vi "Calculate Galvo Control Voltage to Image Size and Max FOV.vi"(8 "Error In":errorcluster, 11 "System Parameters [In]":T1={"Optical Parameters"={"Obj. Focal Length [mm]"=0.0, "Scan Lens EFL[mm]"=0.0, "Tube Lens EFL[mm]"=0.0, "Galvo V Range (+/-)"=0.0, "Galvo Max Half Angle [Deg]"=0.0, "Max Galvo Range[%]"=0.0}, "Vibratome"={"Z Bottom [mm]"=0.0, "Pre Cut Dwell [s]"=0.0, "Blade Frequency [RPM]"=0, "Slice Speed [mm/s]"=0.0, "Post Cut Dwell [s]"=0.0, "Ramp Time [s]"=0.0, "Start X [mm]"=0.0, "Start Y [mm]"=0.0, "Slice Length [mm]"=0.0, "Slice Axis"=enum."Y Axis", "Controller VISA Ref"="COM4", "Blade Frequency [Hz]"=0, "Analog Out Channel"="GalvoCtrl/ao0,GalvoCtrl/ao1", "Pixel Clock Source"="/GalvoCtrl/PFI0"}, "Table Stages"={"X Stage"={"Position"=0.0, "Is.Enabled?"=FALSE, "Is.Connected?"=FALSE, "Device SN"="45876539", "AccelerationMaximum"=0.0, "VelocityMaximum"=0.0, "Acceleration"=0.0, "Velocity"=0.0, "waitTimeout (ms)"=0, "Model"=enum."None", "Is.Homed?"=FALSE, "MOVE"=FALSE}, "Y Stage"={"Position"=0.0, "Is.Enabled?"=FALSE, "Is.Connected?"=FALSE, "Device SN"="45876539", "AccelerationMaximum"=0.0, "VelocityMaximum"=0.0, "Acceleration"=0.0, "Velocity"=0.0, "waitTimeout (ms)"=0, "Model"=enum."None", "Is.Homed?"=FALSE, "MOVE"=FALSE}, "Z Stage"={"Position"=0.0, "Is.Enabled?"=FALSE, "Is.Connected?"=FALSE, "Device SN"="45876539", "AccelerationMaximum"=0.0, "VelocityMaximum"=0.0, "Acceleration"=0.0, "Velocity"=0.0, "waitTimeout (ms)"=0, "Model"=enum."None", "Is.Homed?"=FALSE, "MOVE"=FALSE}}, "Imaging Parameter"={"Raster Scan Direction"=enum."Uni Directional", "Pixel Dwell Time [Clock Cycles]"=0, "Flyback Time [Clock Cycles]"=0, "XY Center [um]"={"X"=1.0, "Y"=1.0}, "Pixel Step Size [um] X"=1.0, "XY Image Size"=enum."256 x 256", "Custom"=FALSE, "Custom Size"={"X"=1, "Y"=1}, "Line Averages"=1, "Pixel Step Size [um] Y"=0.0}, "Galvo HW Parameters"={"Analog Out Channel"="GalvoCtrl/ao0,GalvoCtrl/ao1", "Min Voltage"=-10.0, "Max Voltage"=10.0, "Pixel Clock Source"="/GalvoCtrl/PFI0", "Sample Rate"=1000.0, "Line Clock Out Ch"="GalvoCtrl/port0/line0", "2P ready check"="GalvoCtrl/port0/line0"}, "Alazar parameters"={"Trigger Settings"={"General Trigger Settings"={"Trigger Operation"=0, "Coupling ID"=2, "Range ID"=2, "Delay"=0, "Timeout Ticks"=0, "Mode"=1, "Parameter"=1}, "Trigger Engine 1"={"Trigger Engine"=0, "Source"=2, "Slope"=1, "Level"=140}, "Trigger Engine 2"={"Trigger Engine"=1000, "Source"=4294967295, "Slope"=1, "Level"=2048}}, "Device ID"={"System ID"=1, "Board ID"=1}, "Ch A Input Control"={"Channel"=1, "Coupling"=2, "Range"=10, "Impedance"=2}, "Ch B Input Control"={"Channel"=2, "Coupling"=2, "Range"=10, "Impedance"=2}, "Acq Settings"={"Record Length"=1440, "Offset"=0, "Records Per Buffer"=2048, "Records Count (Records/Acq)"=2147483647, "Window Type"=1, "Footer"=0, "Samples per record"=2048, "Output Format"=257}, "Capture Clock"={"Sample Rate"=100, "Decimation"=0, "Source"=2, "Edge"=0}}, "Mosaic Paramter"={"X Axis"={"Start [mm]"=0.0, "Steps [pts]"=0.0, "End [mm]"=0.0}, "Y Axis"={"Start [mm]"=0.0, "Steps [pts]"=0.0, "End [mm]"=0.0}, "Scan Pattern"=enum."Uni-directional", "Overlap Options"={"Overlap Type"=enum."No Overlap", "Percent Overlap"=0, "Justify"=enum."Start"}}, "Manual Controls"={"Z0"=10.0, "First image height"=0.0, "Data Path"=path "", "Save parameters"={"start pixel"=45, "#pixels to save"=100}, "Center Galvos"=FALSE, "Acquisition mode"=enum."Alazar FFT", "PSOCT Channel"=1, "Save"=FALSE, "AIP rotation angle"=0.0, "ret ds"=FALSE, "Pause?"=FALSE, "Outgoing Mail Server (SMTP)"="smtp.gmail.com", "Email"="", "Password"="", "Carrier 1"=enum."Sprint", "phone number 1"="", "Subject"="", "Message"="", "blocker position"=enum."every two slices", "Carrier 2"=enum."Sprint", "phone number 2"="", "tissue boundary"=FALSE, "Threshold"=0.0}, "Vibratome Axis"={"Start [mm](first cut height)"=45.85, "slice thickness[um]"=2.1, "#slice"=111, "image thickness(um)"=0.0, "#images"=0, "30um?"=FALSE}} {"Manual Controls"."PSOCT Channel" items=["A"=1, "B"=2, "A + B"=3, "C"=4, "A + C"=5, "A + B"=6, "D"=8, "A + D"=9, "B + D"=10, "C + D"=12, "A + B + C + D"=15]; "Alazar parameters"."Capture Clock"."Edge" items=["Rising", "Falling"]; "Alazar parameters"."Capture Clock"."Source" items=["Internal"=1, "Fast External"=2, "Medium External"=3, "Slow External"=4, "External AC"=5, "External DC"=6, "External 10MHz"=7]; "Alazar parameters"."Acq Settings"."Output Format" items=["Float Log"=11, "Float Amp"=10, "U16_LOG"=1, "U16_AMP2"=257, "Real"=3, "Imag"=4]; "Alazar parameters"."Acq Settings"."Footer" items=["FOOTER_NONE", "FOOTER_NPT"]; "Alazar parameters"."Acq Settings"."Window Type" items=["DSP_WINDOW_NONE", "DSP_WINDOW_HANNING", "DSP_WINDOW_HAMMING", "DSP_WINDOW_BLACKMAN", "DSP_WINDOW_BLACKMAN_HARRIS", "DSP_WINDOW_BARTLETT"]; "Alazar parameters"."Ch B Input Control"."Channel" items=["A"=1, "B"=2, "C"=4, "D"=8]; "Alazar parameters"."Ch B Input Control"."Coupling" items=["AC"=1, "DC"=2]; "Alazar parameters"."Ch B Input Control"."Range" items=["20 mV"=1, "40 mV"=2, "50 mV"=3, "80 mV"=4, "100 mV"=5, "200 mV"=6, "400 mV"=7, "500 mV"=8, "800 mV"=9, "1 V"=10, "1.25 V"=33, "2 V"=11, "4 V"=12, "5 V"=13, "8 V"=14, "10 V"=15, "20 V"=16]; "Alazar parameters"."Ch B Input Control"."Impedance" items=["1 MOhm"=1, "50 Ohm"=2, ""=0]; "Alazar parameters"."Ch A Input Control"."Channel" items=["A"=1, "B"=2, "C"=4, "D"=8]; "Alazar parameters"."Ch A Input Control"."Coupling" items=["AC"=1, "DC"=2]; "Alazar parameters"."Ch A Input Control"."Range" items=["20 mV"=1, "40 mV"=2, "50 mV"=3, "80 mV"=4, "100 mV"=5, "200 mV"=6, "400 mV"=7, "500 mV"=8, "800 mV"=9, "1 V"=10, "1.25 V"=33, "2 V"=11, "4 V"=12, "5 V"=13, "8 V"=14, "10 V"=15, "20 V"=16]; "Alazar parameters"."Ch A Input Control"."Impedance" items=["1 MOhm"=1, "50 Ohm"=2, ""=0]; "Alazar parameters"."Trigger Settings"."General Trigger Settings"."Trigger Operation" items=["J", "K", "J OR K", "J AND K", "J XOR K", "J AND NOT K", "NOT J AND K"]; "Alazar parameters"."Trigger Settings"."General Trigger Settings"."Coupling ID" items=["AC"=1, "DC"=2]; "Alazar parameters"."Trigger Settings"."General Trigger Settings"."Range ID" items=["5 V", "1 V", "TTL"]; "Alazar parameters"."Trigger Settings"."Trigger Engine 1"."Trigger Engine" items=["J", "K"]; "Alazar parameters"."Trigger Settings"."Trigger Engine 1"."Source" items=["A", "B", "External", "Disable", "C", "D"]; "Alazar parameters"."Trigger Settings"."Trigger Engine 1"."Slope" items=["Positive"=1, "Negative"=2]; "Alazar parameters"."Trigger Settings"."Trigger Engine 2"."Trigger Engine" items=["J", "K"]; "Alazar parameters"."Trigger Settings"."Trigger Engine 2"."Source" items=["A", "B", "External", "Disable", "C", "D"]; "Alazar parameters"."Trigger Settings"."Trigger Engine 2"."Slope" items=["Positive"=1, "Negative"=2]; "Imaging Parameter"."Pixel Step Size [um] Y" min=0.0 max=10.0 step=0.01; "Imaging Parameter"."Line Averages" min=1 max=30 step=1; "Imaging Parameter"."Flyback Time [Clock Cycles]" max=10 step=1; "Imaging Parameter"."Pixel Step Size [um] X" min=0.0 max=10.0 step=0.01; "Imaging Parameter"."Custom Size"."Y" min=1 max=30 step=1; "Imaging Parameter"."Custom Size"."X" min=1 max=30 step=1; "Imaging Parameter"."XY Center [um]"."Y" min=1.0 max=30.0 step=1.0; "Imaging Parameter"."XY Center [um]"."X" min=1.0 max=30.0 step=1.0; "Imaging Parameter"."Pixel Dwell Time [Clock Cycles]" max=10 step=1}) -> (0 "Error Out":errorcluster, 1 "Max Half FOV (um)":dbl, 2 "Galvo [um/V]":dbl, 3 "System Parameters [Out]":T1={"Optical Parameters"={"Obj. Focal Length [mm]"=0.0, "Scan Lens EFL[mm]"=0.0, "Tube Lens EFL[mm]"=0.0, "Galvo V Range (+/-)"=0.0, "Galvo Max Half Angle [Deg]"=0.0, "Max Galvo Range[%]"=0.0}, "Vibratome"={"Z Bottom [mm]"=0.0, "Pre Cut Dwell [s]"=0.0, "Blade Frequency [RPM]"=0, "Slice Speed [mm/s]"=0.0, "Post Cut Dwell [s]"=0.0, "Ramp Time [s]"=0.0, "Start X [mm]"=0.0, "Start Y [mm]"=0.0, "Slice Length [mm]"=0.0, "Slice Axis"=enum."Y Axis", "Controller VISA Ref"="COM4", "Blade Frequency [Hz]"=0, "Analog Out Channel"="GalvoCtrl/ao0,GalvoCtrl/ao1", "Pixel Clock Source"="/GalvoCtrl/PFI0"}, "Table Stages"={"X Stage"={"Position"=0.0, "Is.Enabled?"=FALSE, "Is.Connected?"=FALSE, "Device SN"="45876539", "AccelerationMaximum"=0.0, "VelocityMaximum"=0.0, "Acceleration"=0.0, "Velocity"=0.0, "waitTimeout (ms)"=0, "Model"=enum."None", "Is.Homed?"=FALSE, "MOVE"=FALSE}, "Y Stage"={"Position"=0.0, "Is.Enabled?"=FALSE, "Is.Connected?"=FALSE, "Device SN"="45876539", "AccelerationMaximum"=0.0, "VelocityMaximum"=0.0, "Acceleration"=0.0, "Velocity"=0.0, "waitTimeout (ms)"=0, "Model"=enum."None", "Is.Homed?"=FALSE, "MOVE"=FALSE}, "Z Stage"={"Position"=0.0, "Is.Enabled?"=FALSE, "Is.Connected?"=FALSE, "Device SN"="45876539", "AccelerationMaximum"=0.0, "VelocityMaximum"=0.0, "Acceleration"=0.0, "Velocity"=0.0, "waitTimeout (ms)"=0, "Model"=enum."None", "Is.Homed?"=FALSE, "MOVE"=FALSE}}, "Imaging Parameter"={"Raster Scan Direction"=enum."Uni Directional", "Pixel Dwell Time [Clock Cycles]"=0, "Flyback Time [Clock Cycles]"=0, "XY Center [um]"={"X"=1.0, "Y"=1.0}, "Pixel Step Size [um] X"=1.0, "XY Image Size"=enum."256 x 256", "Custom"=FALSE, "Custom Size"={"X"=1, "Y"=1}, "Line Averages"=1, "Pixel Step Size [um] Y"=0.0}, "Galvo HW Parameters"={"Analog Out Channel"="GalvoCtrl/ao0,GalvoCtrl/ao1", "Min Voltage"=-10.0, "Max Voltage"=10.0, "Pixel Clock Source"="/GalvoCtrl/PFI0", "Sample Rate"=1000.0, "Line Clock Out Ch"="GalvoCtrl/port0/line0", "2P ready check"="GalvoCtrl/port0/line0"}, "Alazar parameters"={"Trigger Settings"={"General Trigger Settings"={"Trigger Operation"=0, "Coupling ID"=2, "Range ID"=2, "Delay"=0, "Timeout Ticks"=0, "Mode"=1, "Parameter"=1}, "Trigger Engine 1"={"Trigger Engine"=0, "Source"=2, "Slope"=1, "Level"=140}, "Trigger Engine 2"={"Trigger Engine"=1000, "Source"=4294967295, "Slope"=1, "Level"=2048}}, "Device ID"={"System ID"=1, "Board ID"=1}, "Ch A Input Control"={"Channel"=1, "Coupling"=2, "Range"=10, "Impedance"=2}, "Ch B Input Control"={"Channel"=2, "Coupling"=2, "Range"=10, "Impedance"=2}, "Acq Settings"={"Record Length"=1440, "Offset"=0, "Records Per Buffer"=2048, "Records Count (Records/Acq)"=2147483647, "Window Type"=1, "Footer"=0, "Samples per record"=2048, "Output Format"=257}, "Capture Clock"={"Sample Rate"=100, "Decimation"=0, "Source"=2, "Edge"=0}}, "Mosaic Paramter"={"X Axis"={"Start [mm]"=0.0, "Steps [pts]"=0.0, "End [mm]"=0.0}, "Y Axis"={"Start [mm]"=0.0, "Steps [pts]"=0.0, "End [mm]"=0.0}, "Scan Pattern"=enum."Uni-directional", "Overlap Options"={"Overlap Type"=enum."No Overlap", "Percent Overlap"=0, "Justify"=enum."Start"}}, "Manual Controls"={"Z0"=10.0, "First image height"=0.0, "Data Path"=path "", "Save parameters"={"start pixel"=45, "#pixels to save"=100}, "Center Galvos"=FALSE, "Acquisition mode"=enum."Alazar FFT", "PSOCT Channel"=1, "Save"=FALSE, "AIP rotation angle"=0.0, "ret ds"=FALSE, "Pause?"=FALSE, "Outgoing Mail Server (SMTP)"="smtp.gmail.com", "Email"="", "Password"="", "Carrier 1"=enum."Sprint", "phone number 1"="", "Subject"="", "Message"="", "blocker position"=enum."every two slices", "Carrier 2"=enum."Sprint", "phone number 2"="", "tissue boundary"=FALSE, "Threshold"=0.0}, "Vibratome Axis"={"Start [mm](first cut height)"=45.85, "slice thickness[um]"=2.1, "#slice"=111, "image thickness(um)"=0.0, "#images"=0, "30um?"=FALSE}} {"Manual Controls"."PSOCT Channel" items=["A"=1, "B"=2, "A + B"=3, "C"=4, "A + C"=5, "A + B"=6, "D"=8, "A + D"=9, "B + D"=10, "C + D"=12, "A + B + C + D"=15]; "Alazar parameters"."Capture Clock"."Edge" items=["Rising", "Falling"]; "Alazar parameters"."Capture Clock"."Source" items=["Internal"=1, "Fast External"=2, "Medium External"=3, "Slow External"=4, "External AC"=5, "External DC"=6, "External 10MHz"=7]; "Alazar parameters"."Acq Settings"."Output Format" items=["Float Log"=11, "Float Amp"=10, "U16_LOG"=1, "U16_AMP2"=257, "Real"=3, "Imag"=4]; "Alazar parameters"."Acq Settings"."Footer" items=["FOOTER_NONE", "FOOTER_NPT"]; "Alazar parameters"."Acq Settings"."Window Type" items=["DSP_WINDOW_NONE", "DSP_WINDOW_HANNING", "DSP_WINDOW_HAMMING", "DSP_WINDOW_BLACKMAN", "DSP_WINDOW_BLACKMAN_HARRIS", "DSP_WINDOW_BARTLETT"]; "Alazar parameters"."Ch B Input Control"."Channel" items=["A"=1, "B"=2, "C"=4, "D"=8]; "Alazar parameters"."Ch B Input Control"."Coupling" items=["AC"=1, "DC"=2]; "Alazar parameters"."Ch B Input Control"."Range" items=["20 mV"=1, "40 mV"=2, "50 mV"=3, "80 mV"=4, "100 mV"=5, "200 mV"=6, "400 mV"=7, "500 mV"=8, "800 mV"=9, "1 V"=10, "1.25 V"=33, "2 V"=11, "4 V"=12, "5 V"=13, "8 V"=14, "10 V"=15, "20 V"=16]; "Alazar parameters"."Ch B Input Control"."Impedance" items=["1 MOhm"=1, "50 Ohm"=2, ""=0]; "Alazar parameters"."Ch A Input Control"."Channel" items=["A"=1, "B"=2, "C"=4, "D"=8]; "Alazar parameters"."Ch A Input Control"."Coupling" items=["AC"=1, "DC"=2]; "Alazar parameters"."Ch A Input Control"."Range" items=["20 mV"=1, "40 mV"=2, "50 mV"=3, "80 mV"=4, "100 mV"=5, "200 mV"=6, "400 mV"=7, "500 mV"=8, "800 mV"=9, "1 V"=10, "1.25 V"=33, "2 V"=11, "4 V"=12, "5 V"=13, "8 V"=14, "10 V"=15, "20 V"=16]; "Alazar parameters"."Ch A Input Control"."Impedance" items=["1 MOhm"=1, "50 Ohm"=2, ""=0]; "Alazar parameters"."Trigger Settings"."General Trigger Settings"."Trigger Operation" items=["J", "K", "J OR K", "J AND K", "J XOR K", "J AND NOT K", "NOT J AND K"]; "Alazar parameters"."Trigger Settings"."General Trigger Settings"."Coupling ID" items=["AC"=1, "DC"=2]; "Alazar parameters"."Trigger Settings"."General Trigger Settings"."Range ID" items=["5 V", "1 V", "TTL"]; "Alazar parameters"."Trigger Settings"."Trigger Engine 1"."Trigger Engine" items=["J", "K"]; "Alazar parameters"."Trigger Settings"."Trigger Engine 1"."Source" items=["A", "B", "External", "Disable", "C", "D"]; "Alazar parameters"."Trigger Settings"."Trigger Engine 1"."Slope" items=["Positive"=1, "Negative"=2]; "Alazar parameters"."Trigger Settings"."Trigger Engine 2"."Trigger Engine" items=["J", "K"]; "Alazar parameters"."Trigger Settings"."Trigger Engine 2"."Source" items=["A", "B", "External", "Disable", "C", "D"]; "Alazar parameters"."Trigger Settings"."Trigger Engine 2"."Slope" items=["Positive"=1, "Negative"=2]; "Imaging Parameter"."Pixel Step Size [um] Y" min=0.0 max=10.0 step=0.01; "Imaging Parameter"."Line Averages" min=1 max=30 step=1; "Imaging Parameter"."Flyback Time [Clock Cycles]" max=10 step=1; "Imaging Parameter"."Pixel Step Size [um] X" min=0.0 max=10.0 step=0.01; "Imaging Parameter"."Custom Size"."Y" min=1 max=30 step=1; "Imaging Parameter"."Custom Size"."X" min=1 max=30 step=1; "Imaging Parameter"."XY Center [um]"."Y" min=1.0 max=30.0 step=1.0; "Imaging Parameter"."XY Center [um]"."X" min=1.0 max=30.0 step=1.0; "Imaging Parameter"."Pixel Dwell Time [Clock Cycles]" max=10 step=1})   [LabVIEW 2018]
doc: "This is assuming 1:1 magnification between X and Y galvo\n\nChief Ray Angle : The chief ray angle at the back pupil of the objective for the galvo's maximum steering angle.\nOptical Mag: The optical magnification between the galvo and the objective's back pupil\nGalvo: The amount of motion in the object plane per V of control signal on the Galvo.\nMax Half FOV (um) : The maximum object height when the galvos are rotated to max angle."
uses:
  Controls/System Parameters.ctl
  Controls/Optical Parameters.ctl
  Controls/Vibratome Parameters.ctl
  Controls/Translation Stage Parameters.ctl
  Hardware Mfg/Thorlabs Translation Stages/Controls/Translation Stage Cluster.ctl
  Controls/Translation Stage Types.ctl
  Controls/Imaging Parameters.ctl
  Controls/Scan Direction.ctl
  type defines/Alazar parameters.ctl
  Hardware Mfg/AlazarTech SDK/Controls/General Trigger Settings.ctl
  Hardware Mfg/AlazarTech SDK/Controls/Trigger Engine Controls.ctl
  Hardware Mfg/AlazarTech SDK/Controls/Alazar Device ID.ctl
  Hardware Mfg/AlazarTech SDK/Controls/Channel Input Controls.ctl
  Hardware Mfg/AlazarTech SDK/Controls/Alazar Acquisition Settings.ctl
  Hardware Mfg/AlazarTech SDK/Controls/Clock Controls.ctl
  type defines/Manual Controls.ctl
  type defines/FFT parameters.ctl
  type defines/FFT mode.ctl
  type defines/Vibratome Param.ctl
panel:
  out "Chief Ray Angle":dbl
  out "Optical Mag":dbl
  # "X"
  # "X"
  # "X"
  # "X"
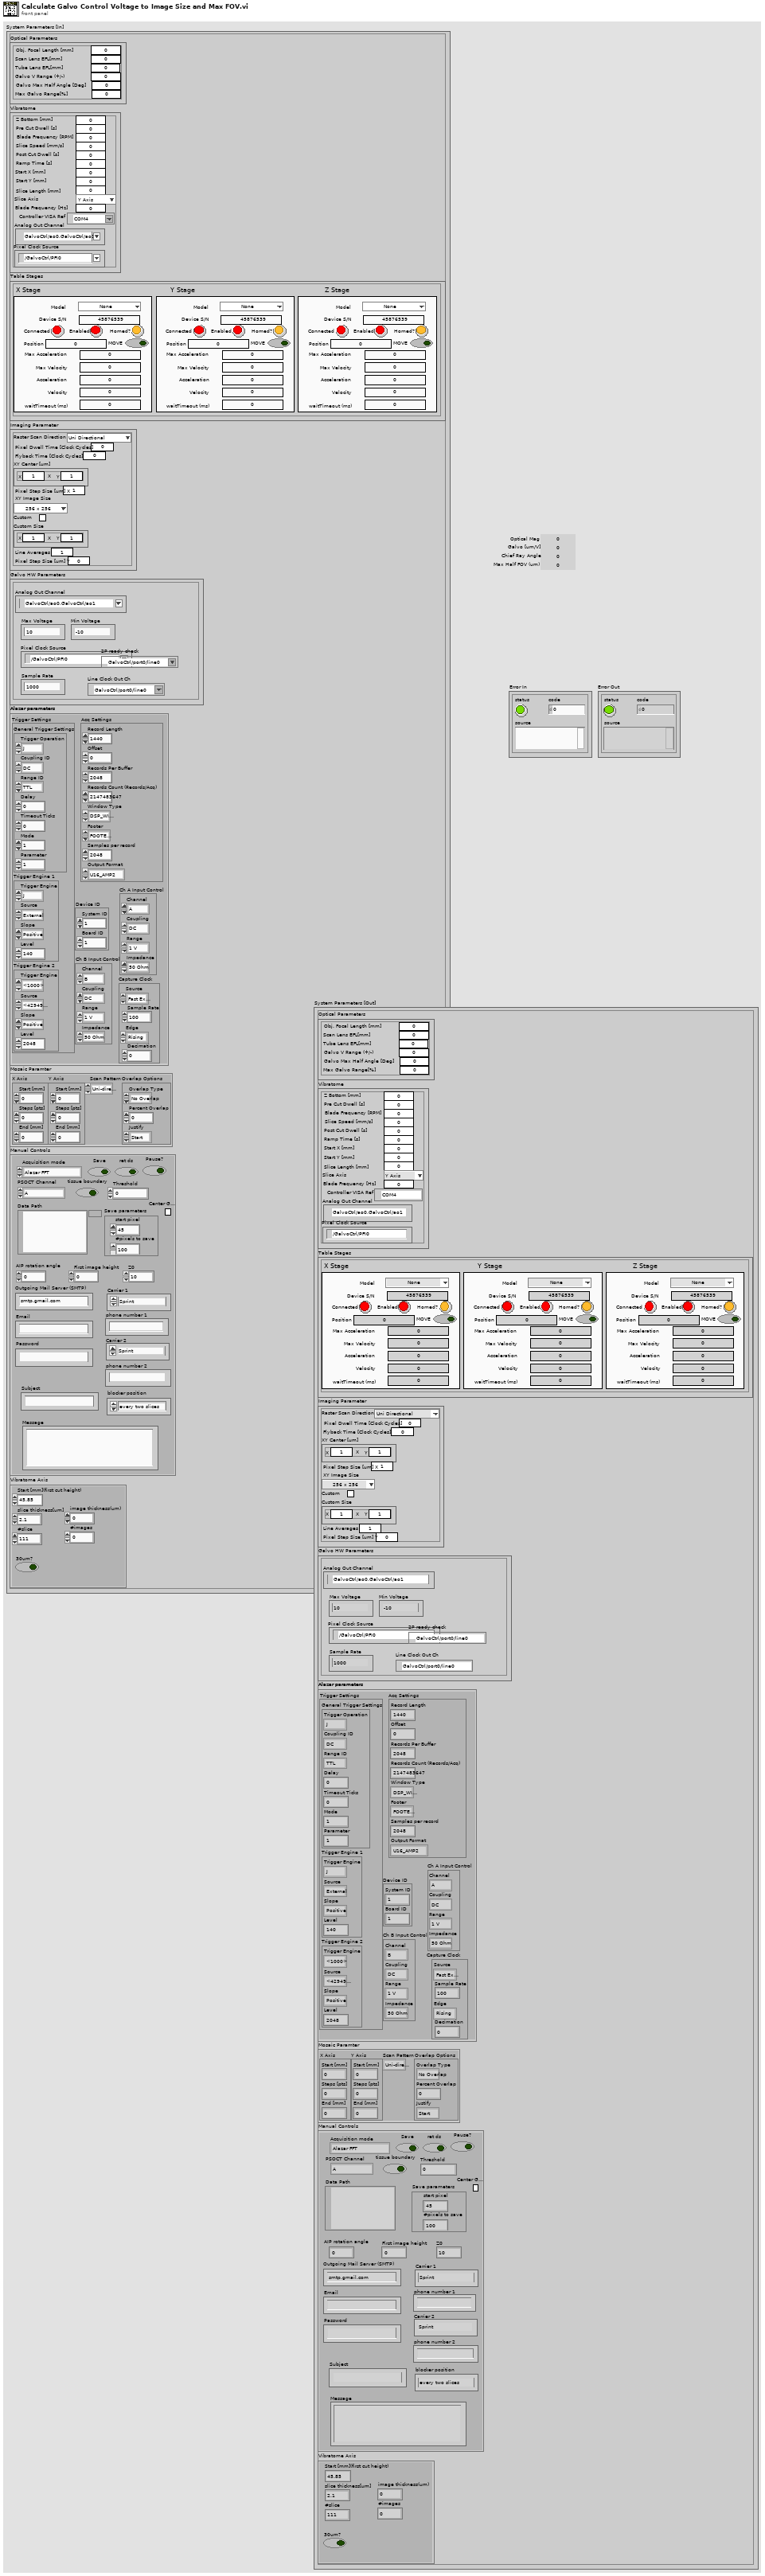
[diagram p1: front panel]
types:
  T1 = typedef "System Parameters.ctl" = cluster{"Optical Parameters":T2, "Vibratome":T3, "Table Stages":T4, "Imaging Parameter":T7, "Galvo HW Parameters":cluster{"Analog Out Channel":tag, "Min Voltage":dbl, "Max Voltage":dbl, "Pixel Clock Source":tag, "Sample Rate":dbl, "Line Clock Out Ch":tag, "2P ready check":tag}, "Alazar parameters":T9, "Mosaic Paramter":cluster{"X Axis":cluster{"Start [mm]":dbl, "Steps [pts]":dbl, "End [mm]":dbl}, "Y Axis":cluster{"Start [mm]":dbl, "Steps [pts]":dbl, "End [mm]":dbl}, "Scan Pattern":enum16{"Uni-directional", "Bi-Directional", "Spiral Out", "Spiral In"}, "Overlap Options":cluster{"Overlap Type":enum16{"No Overlap", "X Only", "Y Only", "X and Y"}, "Percent Overlap":u8, "Justify":enum16{"Start", "Center", "End"}}}, "Manual Controls":T16, "Vibratome Axis":T19}
  T2 = typedef "Optical Parameters.ctl" = cluster{"Obj. Focal Length [mm]":dbl, "Scan Lens EFL[mm]":dbl, "Tube Lens EFL[mm]":dbl, "Galvo V Range (+/-)":dbl, "Galvo Max Half Angle [Deg]":dbl, "Max Galvo Range[%]":dbl}
  T3 = typedef "Vibratome Parameters.ctl" = cluster{"Z Bottom [mm]":dbl, "Pre Cut Dwell [s]":dbl, "Blade Frequency [RPM]":u16, "Slice Speed [mm/s]":dbl, "Post Cut Dwell [s]":dbl, "Ramp Time [s]":dbl, "Start X [mm]":dbl, "Start Y [mm]":dbl, "Slice Length [mm]":dbl, "Slice Axis":enum16{"X Axis", "Y Axis", "Z Axis"}, "Controller VISA Ref":refnum<visa-resource-name>, "Blade Frequency [Hz]":u16, "Analog Out Channel":tag, "Pixel Clock Source":tag}
  T4 = typedef "Translation Stage Parameters.ctl" = cluster{"X Stage":T5, "Y Stage":T5, "Z Stage":T5}
  T5 = typedef "Translation Stage Cluster.ctl" = cluster{"Position":dbl, "Is.Enabled?":bool, "Is.Connected?":bool, "Device SN":string, "AccelerationMaximum":dbl, "VelocityMaximum":dbl, "Acceleration":dbl, "Velocity":dbl, "waitTimeout (ms)":i32, "Model":T6, "Is.Homed?":bool, "MOVE":bool}
  T6 = typedef "Translation Stage Types.ctl" = enum16{"None", "Thorlabs LTS", "Thorlabs MLJ"}
  T7 = typedef "Imaging Parameters.ctl" = cluster{"Raster Scan Direction":T8, "Pixel Dwell Time [Clock Cycles]":u16, "Flyback Time [Clock Cycles]":u16, "XY Center [um]":cluster{"X":dbl, "Y":dbl}, "Pixel Step Size [um] X":dbl, "XY Image Size":enum16{"32 x 32", "64 x 64", "128 x 128", "256 x 256", "512 x 512", "1024 x 1024", "2048 x 2048"}, "Custom":bool, "Custom Size":cluster{"X":u16, "Y":u16}, "Line Averages":u8, "Pixel Step Size [um] Y":dbl}
  T8 = typedef "Scan Direction.ctl" = enum16{"Uni Directional", "Bi Directional", "None"}
  T9 = typedef "Alazar parameters.ctl" = cluster{"Trigger Settings":cluster{"General Trigger Settings":T10, "Trigger Engine 1":T11, "Trigger Engine 2":T11}, "Device ID":T12, "Ch A Input Control":T13, "Ch B Input Control":T13, "Acq Settings":T14, "Capture Clock":T15}
  T10 = typedef "General Trigger Settings.ctl" = cluster{"Trigger Operation":u32, "Coupling ID":u32, "Range ID":u32, "Delay":u32, "Timeout Ticks":u32, "Mode":u32, "Parameter":u32}
  T11 = typedef "Trigger Engine Controls.ctl" = cluster{"Trigger Engine":u32, "Source":u32, "Slope":u32, "Level":u32}
  T12 = typedef "Alazar Device ID.ctl" = cluster{"System ID":u32, "Board ID":u32}
  T13 = typedef "Channel Input Controls.ctl" = cluster{"Channel":u8, "Coupling":u32, "Range":u32, "Impedance":u32}
  T14 = typedef "Alazar Acquisition Settings.ctl" = cluster{"Record Length":u32, "Offset":u32, "Records Per Buffer":u32, "Records Count (Records/Acq)":u32, "Window Type":u32, "Footer":u32, "Samples per record":u32, "Output Format":u32}
  T15 = typedef "Clock Controls.ctl" = cluster{"Sample Rate":u32, "Decimation":u32, "Source":u32, "Edge":u32}
  T16 = typedef "Manual Controls.ctl" = cluster{"Z0":dbl, "First image height":dbl, "Data Path":path, "Save parameters":T17, "Center Galvos":bool, "Acquisition mode":T18, "PSOCT Channel":u32, "Save":bool, "AIP rotation angle":dbl, "ret ds":bool, "Pause?":bool, "Outgoing Mail Server (SMTP)":string, "Email":string, "Password":string, "Carrier 1":enum16{"T-Mobile", "AT&T", "Verizon", "Sprint"}, "phone number 1":string, "Subject":string, "Message":string, "blocker position":enum16{"every two slices", "Nat slices", "None"}, "Carrier 2":enum16{"T-Mobile", "AT&T", "Verizon", "Sprint"}, "phone number 2":string, "tissue boundary":bool, "Threshold":sgl}
  T17 = typedef "FFT parameters.ctl" = cluster{"start pixel":i32, "#pixels to save":i32}
  T18 = typedef "FFT mode.ctl" = enum16{"ThorOCT B line", "ThorOCT Spectral", "ThorOCT FFT", "Alazar B line", "Alazar FFT", "GPU FFT", "Alazar Spectral", "Simulation", "auto adjust focus", "Save all"}
  T19 = typedef "Vibratome Param.ctl" = cluster{"Start [mm](first cut height)":dbl, "slice thickness[um]":dbl, "#slice":u16, "image thickness(um)":dbl, "#images":u16, "30um?":bool}
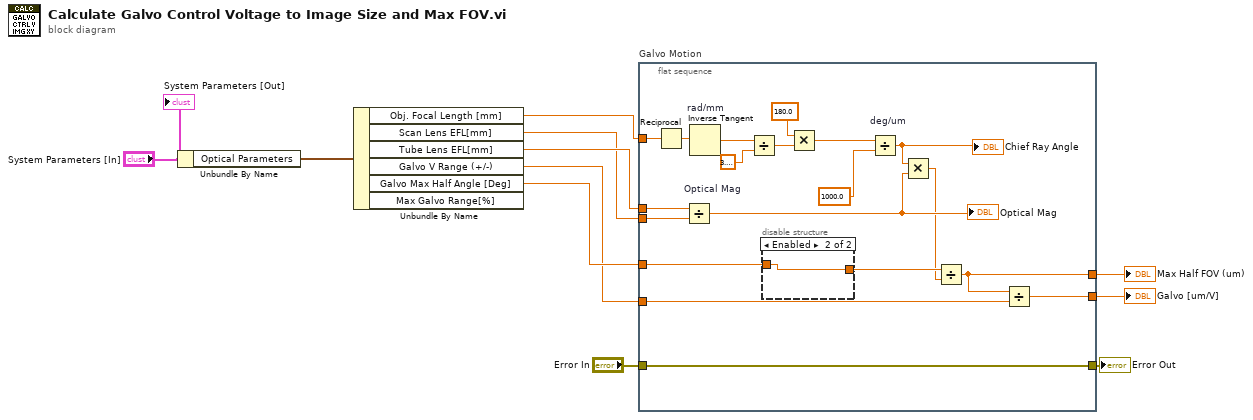
[diagram p0: block diagram]
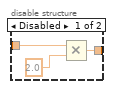
[diagram p2: hidden frame]
diagram:
  n1 = Unbundle By Name("System Parameters [In]") -> ("Optical Parameters"=w10:T2)
  n2 = Unbundle By Name(w10) -> ("Obj. Focal Length [mm]"=w7:dbl, "Scan Lens EFL[mm]"=w5:dbl, "Tube Lens EFL[mm]"=w6:dbl, "Galvo V Range (+/-)"=w8:dbl, "Galvo Max Half Angle [Deg]"=w9:dbl)  [unwired: 1 out]
  n3 = flat-sequence "Galvo Motion" {
    tunnel: w9 -> [w15]
    tunnel: w8 -> [w14]
    tunnel: w7 -> [w27]
    tunnel: w6 -> [w26]
    tunnel: w5 -> [w25]
    tunnel: "Error In" -> [w24]
    tunnel: [w24] -> w3
    tunnel: [w12] -> w2
    tunnel: [w13] -> w1
    frame #0 {
      n4 = Reciprocal(x=w27) -> (1/x=w28:dbl)
      n5 = Divide "Optical Mag"(x=w26, y=w25) -> (x/y=w18:dbl)
      "Optical Mag" <- w18
      n6 = Inverse Tangent "rad/mm"(1:w28) -> (0:w29:dbl)
      n7 = Divide(x=w29, y=3.141592653589793) -> (x/y=w23:dbl)
      n8 = disable-structure shown="Enabled" {
        disable-tunnel: [w32 w34] -> w17
        disable-tunnel: w15 -> [w31 w34]
        frame Disabled {
          n9 = Multiply(x=w31, y=2.0 ("x")) -> (x*y=w32:dbl)
        }
        frame Enabled {
        }
      }
      n10 = Multiply(x=180.0, y=w23) -> (x*y=w20:dbl)
      n11 = Divide "deg/um"(x=w20, y=1000.0) -> (x/y=w19:dbl)
      "Chief Ray Angle" <- w19
      n12 = Multiply(x=w19, y=w18) -> (x*y=w16:dbl)
      n13 = Divide(x=w17, y=w16) -> (x/y=w12:dbl)
      n14 = Divide(x=w12, y=w14) -> (x/y=w13:dbl)
    }
  }
  "Galvo [um/V]" <- w1
  "Max Half FOV (um)" <- w2
  "System Parameters [Out]" <- "System Parameters [In]"
  "Error Out" <- w3
